vi "Constants.vi"() -> ()   [LabVIEW 2018]
panel:
  in  "ElevatorSetpoints":dbl[](array[numeric])=[13.5, 40.5, 94.0, 83.0]
  in  "Track Width":dbl=29.0
  in  "CenterRotOffset":dbl=19.5
  in  "Height":dbl=38.5
  in  "Width":dbl=33.0
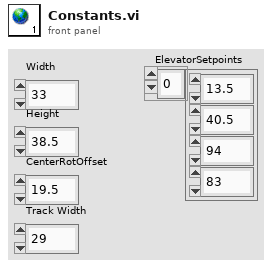
[diagram p1: front panel]
diagram:
